vi "Util_Trajectory_to_XY.vi"(11 "TRAJECTORY":T1 {"TotalTImeSecs" format="%20.3f"}) -> (3 "outArrayXY":cluster{dbl[], dbl[]})   [LabVIEW 2019]
doc: "This is a convience function to convert the X, Y portions of a PoseWithCurvature array into arrays of X,Y for charting."
uses:
  <vilib>/Rock Robotics/WPI/ThirdParty/JAS_Junk/TrajLib/TRANSLATION2D.ctl
  <vilib>/Rock Robotics/WPI/ThirdParty/JAS_Junk/TrajLib/Trajectory_Library.lvlib
  <vilib>/Rock Robotics/WPI/ThirdParty/JAS_Junk/TrajLib/ROTATION2D.ctl
  <vilib>/Rock Robotics/WPI/ThirdParty/JAS_Junk/TrajLib/POSE2D.ctl
  <vilib>/Rock Robotics/WPI/ThirdParty/JAS_Junk/TrajLib/TRAJ_STATE.ctl
  <vilib>/Rock Robotics/WPI/ThirdParty/JAS_Junk/TrajLib/TRAJECTORY.ctl
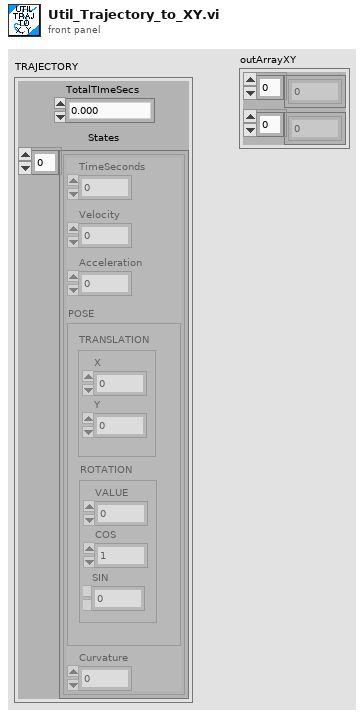
[diagram p1: front panel]
types:
  T1 = typedef "Trajectory_Library.lvlib/TRAJECTORY.ctl" = cluster{"TotalTImeSecs":dbl, "States":T2[]}
  T2 = typedef "Trajectory_Library.lvlib/TRAJ_STATE.ctl" = cluster{"TimeSeconds":dbl, "Velocity":dbl, "Acceleration":dbl, "POSE":T3, "Curvature":dbl}
  T3 = typedef "Trajectory_Library.lvlib/POSE2D.ctl" = cluster{"TRANSLATION":T4, "ROTATION":T5}
  T4 = typedef "Trajectory_Library.lvlib/TRANSLATION2D.ctl" = cluster{"X":dbl, "Y":dbl}
  T5 = typedef "Trajectory_Library.lvlib/ROTATION2D.ctl" = cluster{"VALUE":dbl, "COS":dbl, "SIN":dbl}
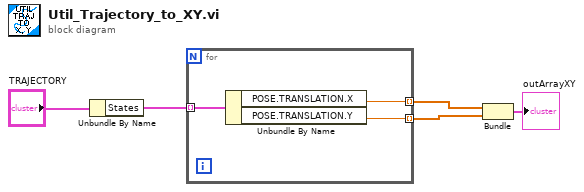
[diagram p0: block diagram]
diagram:
  n1 = Unbundle By Name("TRAJECTORY") -> ("States"=w1:T2[])
  n2 = for {
    tunnel: [w8] -> w4 mode=indexing
    tunnel: [w7] -> w5 mode=indexing
    tunnel: w1 -> [w6] mode=indexing
    n3 = Unbundle By Name(w6) -> ("POSE.TRANSLATION.X"=w8:dbl, "POSE.TRANSLATION.Y"=w7:dbl)
  }
  n4 = Bundle(w4, w5) -> (→"outArrayXY":cluster{dbl[], dbl[]})  [unwired: 1 in]
